vi "Pv.vi"() -> ()   [LabVIEW 2011]
panel:
  in  "Q":dbl
  out "W":dbl
  out "VL":dbl
  in  "Zigmae":dbl[](array[numeric])
  in  "Vr/Wr":dbl[](array[numeric])
  in  "Kp2":dbl
  in  "Kp1":dbl
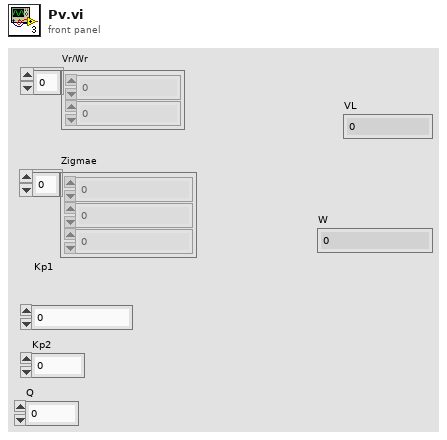
[diagram p1: front panel]
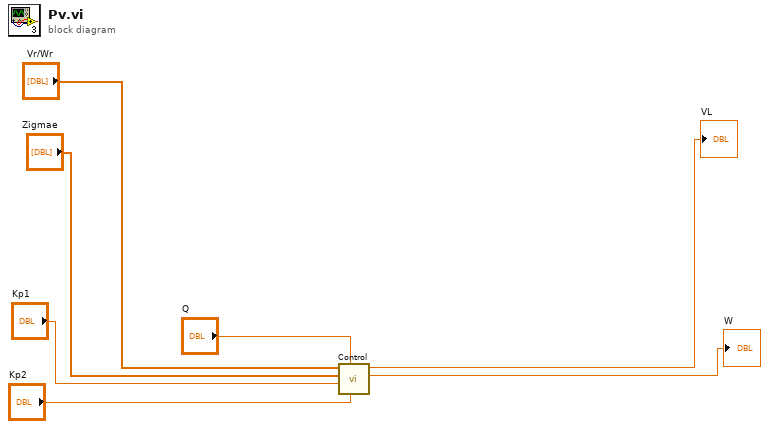
[diagram p0: block diagram]
diagram:
  n1 = call "Control.vi"("Kp2"="Kp2", "Q"="Q", "Kp1"="Kp1", "Zigmae"="Zigmae", "Vr/Wr"="Vr/Wr") -> ("Numeric"=→"W":dbl, "Numeric 2"=→"VL":dbl)  [unwired: 5 in]
